vi "Update Patterns Array.vi"(8 "error in (no error)":errorcluster, 9 "Old Num of Parabolas":u16, 10 "Num of Parabolas":u16, 11 "GUI in":refnum<class "GUI.lvclass">) -> (0 "error out":errorcluster, 3 "GUI out":refnum<class "GUI.lvclass">)   [LabVIEW 2020, in "GUI.lvlib" / "GUI.lvclass"]
uses:
  GUI.lvclass
  GUI.lvclass/GUI.ctl
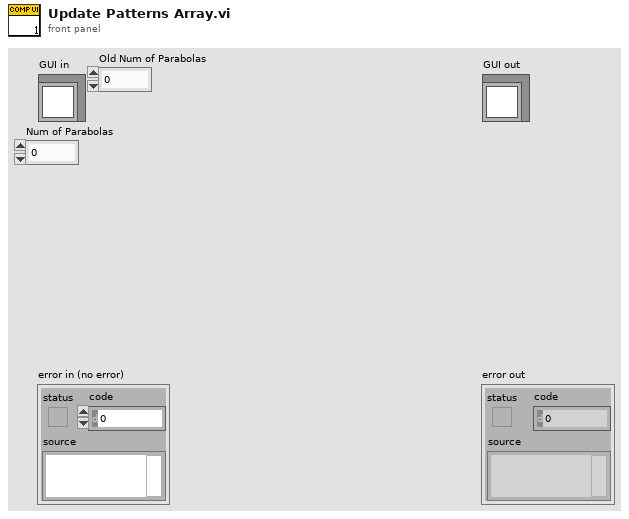
[diagram p1: front panel]
types:
  T1 = typedef "Task selection df.ctl" = cluster{"Task Type Select":enum32{"Frequency Task", "Scanning Task"}, "Input Select Type":enum32{"Force Input", "Movement Input"}, "Collect EMG?":bool, "Collect acceleration?":bool, "EMG Rate":u16, "Acceleration Rate":u16}
  T2 = typedef "Automate df.ctl" = cluster{"Automate?":bool, "Num Parabs":u16, "Patterns Array":u8[][], "Phase Array":i32[][]}
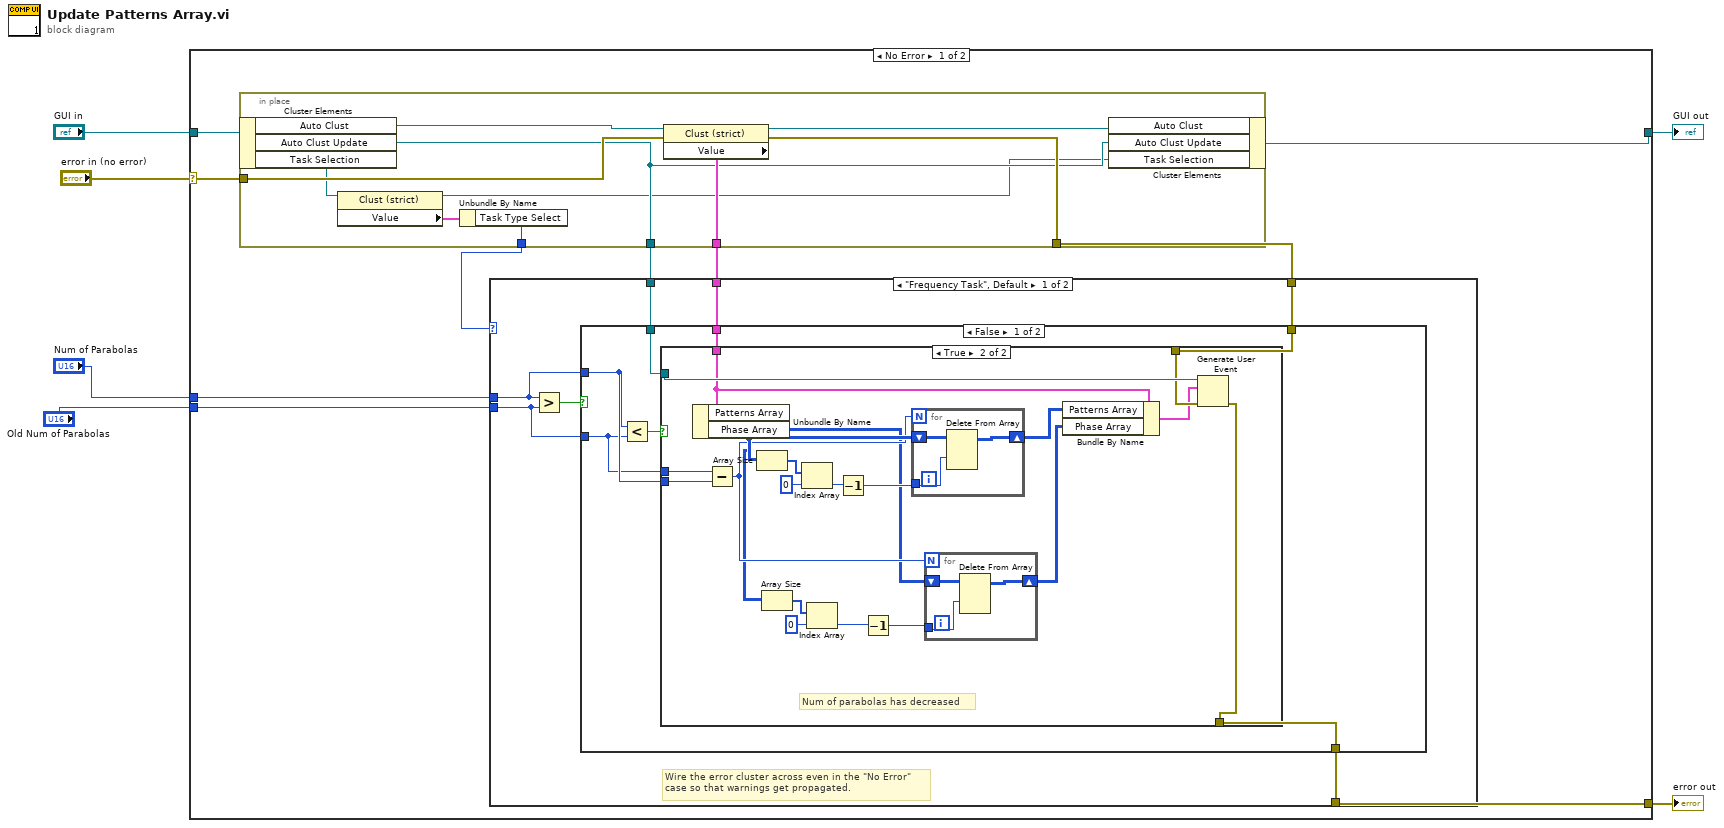
[diagram p0: block diagram]
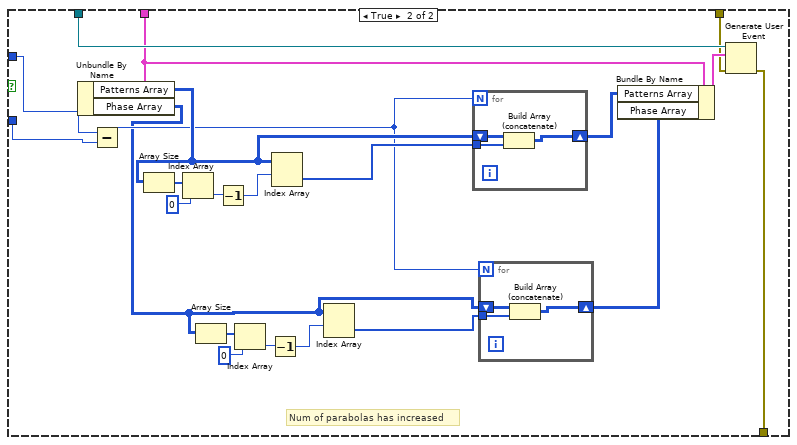
[diagram p3: hidden frame]
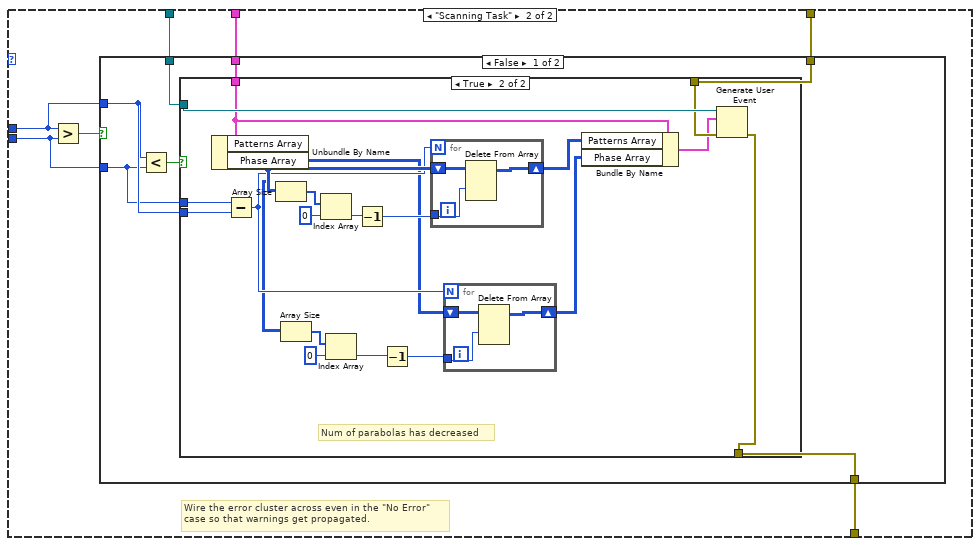
[diagram p4: hidden frame]
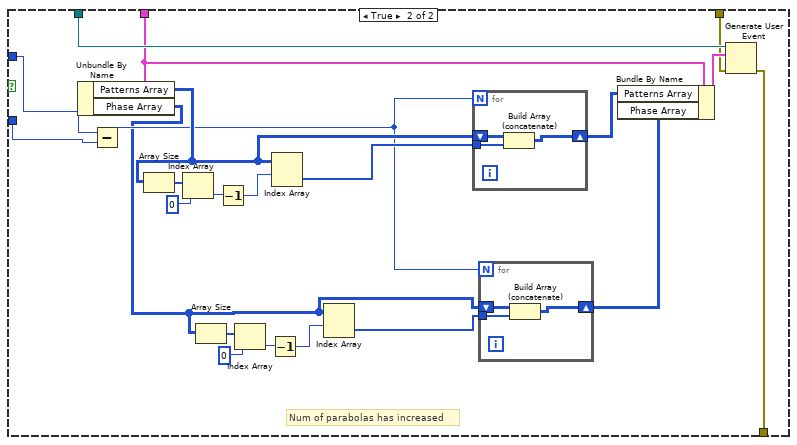
[diagram p6: hidden frame]
diagram:
  n1 = case shown="No Error" "error in (no error)" {
    selector: "error in (no error)" -> [w14 w166]
    tunnel: [w10 w166] -> w5
    tunnel: [w15 w165] -> w3
    tunnel: "GUI in" -> [w16 w165]
    tunnel: "Old Num of Parabolas" -> [w8 _]
    tunnel: "Num of Parabolas" -> [w9 _]
    frame No Error {
      n2 = in-place {
        in-place-border: w14 -> [w163]
        in-place-border: [w159] -> w13
        in-place-border: [w161] -> w12
        in-place-border: [w160] -> w11
        in-place-border: [w156] -> w7
        n3 = in-place-cluster #1(w16) -> ("Auto Clust"=w164:refnum<vi>, "Auto Clust Update"=w159:refnum<user-event>, "Task Selection"=w158:refnum<vi>)
        n4 = property class="Clust (strict)"(reference=w158) -> (reference out=w155:refnum<vi>, "Value"=w157:T1)  [unwired: 1 in, 1 out]
        n5 = Unbundle By Name(w157) -> ("Task Type Select"=w156:enum32{"Frequency Task", "Scanning Task"})
        n6 = property class="Clust (strict)"(reference=w164, error in=w163) -> (reference out=w162:refnum<vi>, error out=w160:errorcluster, "Value"=w161:T2)
        n7 = in-place-cluster #1("Auto Clust"=w162, "Auto Clust Update"=w159, "Task Selection"=w155) -> (w15:refnum<class "GUI.lvclass">)
      }
      n8 = case shown="\"Frequency Task\", Default" w7 {
        tunnel: w13 -> [w22 w91]
        tunnel: w12 -> [w21 w90]
        tunnel: w11 -> [w20 w89]
        tunnel: [w19 w88] -> w10
        tunnel: w9 -> [w18 w87]
        tunnel: w8 -> [w17 w86]
        frame "Frequency Task", Default {
          # "Wire the error cluster across even in the \"No Error\"\ncase so that warnings get propagated."
          n9 = Greater?(x=w18, y=w17) -> (0:w23:bool)
          n10 = case shown="False" w23 {
            tunnel: w18 -> [w25 w66]
            tunnel: w17 -> [w24 w67]
            tunnel: w22 -> [w27 w74]
            tunnel: w21 -> [w26 w72]
            tunnel: w20 -> [w29 w69]
            tunnel: [w28 w68] -> w19
            frame False {
              n11 = Less?(x=w25, y=w24) -> (x < y?=w30:bool)
              n12 = case shown="True" w30 {
                tunnel: w29 -> [w31 w50]
                tunnel: [w31 w41] -> w28
                tunnel: w27 -> [_ w51]
                tunnel: w26 -> [_ w44]
                tunnel: w25 -> [_ w40]
                tunnel: w24 -> [_ w39]
                frame False {
                  # "no change in number of parabolas"
                }
                frame True {
                  # "Num of parabolas has decreased"
                  n13 = Unbundle By Name(w44) -> ("Patterns Array"=w46:u8[][], "Phase Array"=w32:i32[][])
                  n14 = Subtract(x=w39, y=w40) -> (x-y=w34:u16)
                  n15 = Array Size(array=w46) -> (size(s)=w49:i32[])
                  n16 = Array Size(array=w32) -> (size(s)=w38:i32[])
                  n17 = Index Array(array=w49, index=0) -> (element=w47:i32)
                  n18 = Index Array(array=w38, index=0) -> (element=w36:i32)
                  n19 = Decrement(x=w47) -> (x-1=w45:i32)
                  n20 = Decrement(x=w36) -> (x-1=w35:i32)
                  n21 = for {
                    N: w34 -> [_]
                    tunnel: w45 -> [w56]
                    shift-right: [w55] -> w43
                    shift-left: w46 -> [w57]
                    n22 = Delete From Array(array=w57, index (row)=w56) -> (array with subset deleted=w55:u8[][])  [unwired: 2 in, 1 out]
                  }
                  n23 = for {
                    N: w34 -> [_]
                    tunnel: w35 -> [w53]
                    shift-right: [w52] -> w33
                    shift-left: w32 -> [w54]
                    n24 = Delete From Array(array=w54, index (row)=w53) -> (array with subset deleted=w52:i32[][])  [unwired: 2 in, 1 out]
                  }
                  n25 = Bundle By Name(cluster=w44, "Patterns Array"=w43, "Phase Array"=w33) -> (w42:T2)
                  n26 = Generate User Event(user event=w51, event data cluster=w42, error in=w50) -> (error out=w41:errorcluster)  [unwired: 1 in, 1 out]
                }
              }
            }
            frame True {
              # "Num of parabolas has increased"
              n27 = Unbundle By Name(w72) -> ("Patterns Array"=w73:u8[][], "Phase Array"=w58:i32[][])
              n28 = Subtract(x=w66, y=w67) -> (x-y=w60:u16)
              n29 = Array Size(array=w73) -> (size(s)=w79:i32[])
              n30 = Index Array(array=w79, index=0) -> (element=w77:i32)
              n31 = Array Size(array=w58) -> (size(s)=w65:i32[])
              n32 = Decrement(x=w77) -> (x-1=w76:i32)
              n33 = Index Array(array=w65, index=0) -> (element=w63:i32)
              n34 = Decrement(x=w63) -> (x-1=w62:i32)
              n35 = Index Array(array=w73, index (row)=w76) -> (element=w75:u8[])  [unwired: 1 in]
              n36 = Index Array(array=w58, index (row)=w62) -> (element=w61:i32[])  [unwired: 1 in]
              n37 = for {
                N: w60 -> [_]
                tunnel: w75 -> [w85]
                shift-right: [w83] -> w70
                shift-left: w73 -> [w84]
                n38 = Build Array (concatenate)(w84, w85) -> (w83:u8[][])
              }
              n39 = for {
                N: w60 -> [_]
                tunnel: w61 -> [w82]
                shift-right: [w80] -> w59
                shift-left: w58 -> [w81]
                n40 = Build Array (concatenate)(w81, w82) -> (w80:i32[][])
              }
              n41 = Bundle By Name(cluster=w72, "Patterns Array"=w70, "Phase Array"=w59) -> (w71:T2)
              n42 = Generate User Event(user event=w74, event data cluster=w71, error in=w69) -> (error out=w68:errorcluster)  [unwired: 1 in, 1 out]
            }
          }
        }
        frame "Scanning Task" {
          # "Wire the error cluster across even in the \"No Error\"\ncase so that warnings get propagated."
          n43 = Greater?(x=w87, y=w86) -> (0:w92:bool)
          n44 = case shown="False" w92 {
            tunnel: w87 -> [w94 w135]
            tunnel: w86 -> [w93 w136]
            tunnel: w91 -> [w96 w143]
            tunnel: w90 -> [w95 w141]
            tunnel: w89 -> [w98 w138]
            tunnel: [w97 w137] -> w88
            frame False {
              n45 = Less?(x=w94, y=w93) -> (x < y?=w99:bool)
              n46 = case shown="True" w99 {
                tunnel: w98 -> [w100 w119]
                tunnel: [w100 w110] -> w97
                tunnel: w96 -> [_ w120]
                tunnel: w95 -> [_ w113]
                tunnel: w94 -> [_ w109]
                tunnel: w93 -> [_ w108]
                frame False {
                  # "no change in number of parabolas"
                }
                frame True {
                  # "Num of parabolas has decreased"
                  n47 = Unbundle By Name(w113) -> ("Patterns Array"=w115:u8[][], "Phase Array"=w101:i32[][])
                  n48 = Subtract(x=w108, y=w109) -> (x-y=w103:u16)
                  n49 = Array Size(array=w115) -> (size(s)=w118:i32[])
                  n50 = Array Size(array=w101) -> (size(s)=w107:i32[])
                  n51 = Index Array(array=w118, index=0) -> (element=w116:i32)
                  n52 = Index Array(array=w107, index=0) -> (element=w105:i32)
                  n53 = Decrement(x=w116) -> (x-1=w114:i32)
                  n54 = Decrement(x=w105) -> (x-1=w104:i32)
                  n55 = for {
                    N: w103 -> [_]
                    tunnel: w114 -> [w125]
                    shift-right: [w124] -> w112
                    shift-left: w115 -> [w126]
                    n56 = Delete From Array(array=w126, index (row)=w125) -> (array with subset deleted=w124:u8[][])  [unwired: 2 in, 1 out]
                  }
                  n57 = for {
                    N: w103 -> [_]
                    tunnel: w104 -> [w122]
                    shift-right: [w121] -> w102
                    shift-left: w101 -> [w123]
                    n58 = Delete From Array(array=w123, index (row)=w122) -> (array with subset deleted=w121:i32[][])  [unwired: 2 in, 1 out]
                  }
                  n59 = Bundle By Name(cluster=w113, "Patterns Array"=w112, "Phase Array"=w102) -> (w111:T2)
                  n60 = Generate User Event(user event=w120, event data cluster=w111, error in=w119) -> (error out=w110:errorcluster)  [unwired: 1 in, 1 out]
                }
              }
            }
            frame True {
              # "Num of parabolas has increased"
              n61 = Unbundle By Name(w141) -> ("Patterns Array"=w142:u8[][], "Phase Array"=w127:i32[][])
              n62 = Subtract(x=w135, y=w136) -> (x-y=w129:u16)
              n63 = Array Size(array=w142) -> (size(s)=w148:i32[])
              n64 = Index Array(array=w148, index=0) -> (element=w146:i32)
              n65 = Array Size(array=w127) -> (size(s)=w134:i32[])
              n66 = Decrement(x=w146) -> (x-1=w145:i32)
              n67 = Index Array(array=w134, index=0) -> (element=w132:i32)
              n68 = Decrement(x=w132) -> (x-1=w131:i32)
              n69 = Index Array(array=w142, index (row)=w145) -> (element=w144:u8[])  [unwired: 1 in]
              n70 = Index Array(array=w127, index (row)=w131) -> (element=w130:i32[])  [unwired: 1 in]
              n71 = for {
                N: w129 -> [_]
                tunnel: w144 -> [w154]
                shift-right: [w152] -> w139
                shift-left: w142 -> [w153]
                n72 = Build Array (concatenate)(w153, w154) -> (w152:u8[][])
              }
              n73 = for {
                N: w129 -> [_]
                tunnel: w130 -> [w151]
                shift-right: [w149] -> w128
                shift-left: w127 -> [w150]
                n74 = Build Array (concatenate)(w150, w151) -> (w149:i32[][])
              }
              n75 = Bundle By Name(cluster=w141, "Patterns Array"=w139, "Phase Array"=w128) -> (w140:T2)
              n76 = Generate User Event(user event=w143, event data cluster=w140, error in=w138) -> (error out=w137:errorcluster)  [unwired: 1 in, 1 out]
            }
          }
        }
      }
    }
    frame Error {
    }
  }
  "error out" <- w5
  "GUI out" <- w3
